vi "Export dat - I-V.vi"(8 "Error In":errorcluster, 9 "Workspace":path, 11 "IV measurement":T1={"Name"="", "Comment"="", "Time"=timestamp(0 s since 1904-01-01), "Folder"=path "", "IV properties"={"T"=0.0, "Vstart"=-0.5, "Vstop"=0.5, "Vpoints"=10.0, "Settling"=0.01, "I limit"=0.1, "Log mapping"=FALSE, "Averaging"=0.0}, "GUID"=""} {"IV properties"."Settling" min=0.0 max=65535.0}) -> (0 "Error Out":errorcluster)   [LabVIEW 2019]
doc: "Handles export of a I-V measurement to a .dat file, displays a GUI window"
uses:
  Type defs/IV measurement Type Def.ctl
  Type defs/IV properties Type Def.ctl
  <vilib>/Utility/sysdir.llb/System Directory Type.ctl
  <vilib>/Utility/file.llb/Write Delimited Spreadsheet (string).vi
  <vilib>/Utility/file.llb/Write Delimited Spreadsheet (DBL).vi
panel:
  out "String":string
  in  "Path":path caption="Export file as:"
  in  "Export":bool
  in  "Cancel":bool
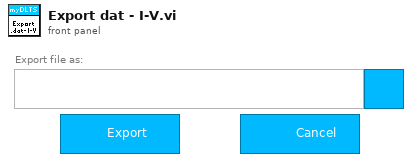
[diagram p1: front panel]
types:
  T1 = typedef "IV measurement Type Def.ctl" = cluster{"Name":string, "Comment":string, "Time":timestamp, "Folder":path, "IV properties":T2, "GUID":string}
  T2 = typedef "IV properties Type Def.ctl" = cluster{"T":dbl[unit], "Vstart":dbl[unit], "Vstop":dbl[unit], "Vpoints":dbl, "Settling":dbl[unit], "I limit":dbl[unit], "Log mapping":bool, "Averaging":dbl}
  T3 = enum32{"existing file", "new file", "new or existing file", "existing dir", "new dir", "new or existing dir", "existing file (use LLBs)", "new file (use LLBs)", "new or existing file (use LLBs)", "new or existing file or directory (use LLBs)", "existing dir (use LLBs)", "new dir (use LLBs)", "new or existing dir (use LLBs)", "existing file or dir", "new file or dir", "new or existing file or dir", "existing file or dir (use LLBs)", "new file or dir (use LLBs)"}
  T4 = typedef "System Directory Type.ctl" = i32
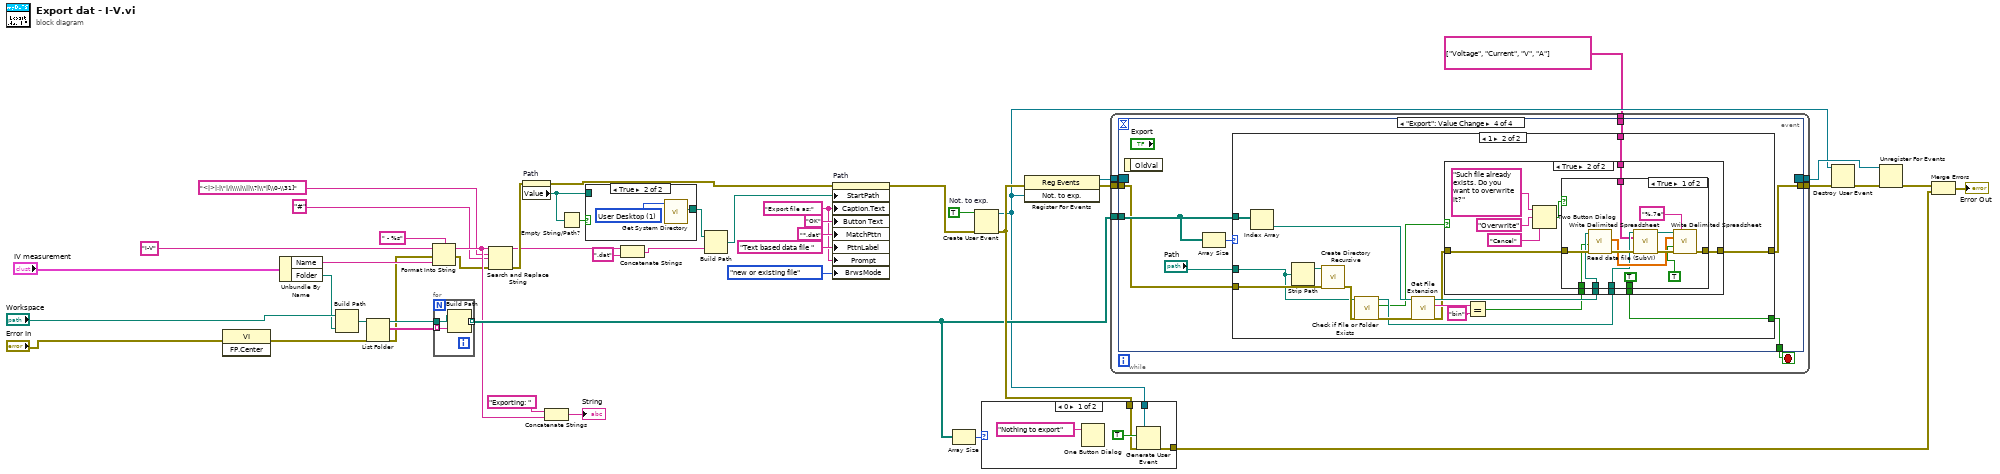
[diagram p0: block diagram]
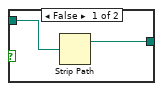
[diagram p2: hidden frame]
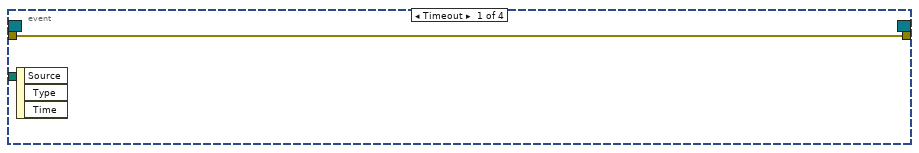
[diagram p4: hidden frame]
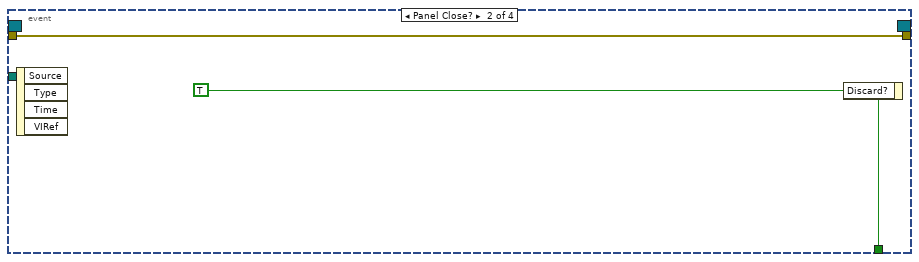
[diagram p5: hidden frame]
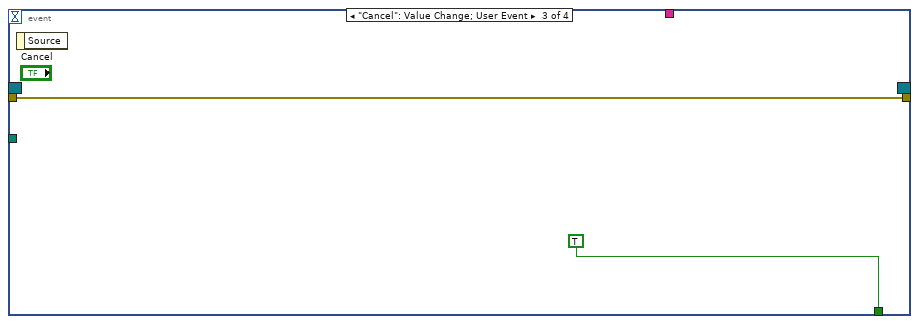
[diagram p6: hidden frame]
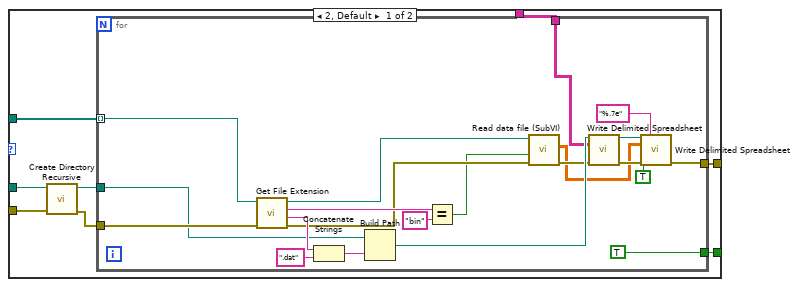
[diagram p7: hidden frame]
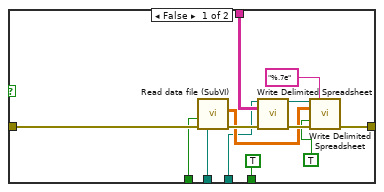
[diagram p8: hidden frame]
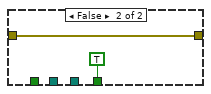
[diagram p9: hidden frame]
diagram:
  w15 = "Export file as:"
  w45 = TRUE  # Not. to exp.
  n1 = invoke class="VI" method="FP.Center"(error in="Error In") -> (error out=w3:errorcluster)  [unwired: 2 in, 2 out]
  n2 = Unbundle By Name("IV measurement") -> ("Name"=w10:string, "Folder"=w20:path)
  n3 = Build Path(base path="Workspace", name or relative path=w20) -> (appended path=w13:path)
  n4 = List Folder(path=w13, error in=w3) -> (path out=w12:path, filenames=w19:string[], error out=w5:errorcluster)  [unwired: 2 in, 1 out]
  n5 = Format Into String(format string=" - %s", initial string="I-V", error in=w5, w10) -> (resulting string=w32:string, error out=w9:errorcluster)
  n6 = for {
    tunnel: w12 -> [w50]
    tunnel: [w49] -> w40 mode=indexing
    tunnel: w19 -> [w48] mode=indexing
    n7 = Build Path(base path=w50, name or relative path=w48) -> (appended path=w49:path)
  }
  n8 = Search and Replace String(input string=w32, search string="<|>|:|\"|/|\\\\|\\||\\?|\\*|[\\0-\\31]", replace string="#" ("replace string (\"\")"), error in=w9) -> (result string=w8:string, error out=w11:errorcluster)  [unwired: 4 in, 2 out]
  n9 = property on="Path" class="Path"(error in=w11) -> (error out=w21:errorcluster, "Value"=w27:path)  [unwired: 1 in, 1 out]
  n10 = Concatenate Strings("Exporting: " ("string"), w32) -> (→"String":string)
  n11 = Empty String/Path?(string/path=w27) -> (empty?=w28:bool)
  n12 = case shown="True" w28 {
    tunnel: w27 -> [w52 _]
    tunnel: [w51 w53] -> w23
    frame False {
      n13 = Strip Path(path=w52) -> (stripped path=w51:path)  [unwired: 1 out]
    }
    frame True {
      w54 = T4 1 items=["User Home"=0, "User Desktop"=1, "User Documents"=2, "User Application Data"=3, "User Preferences"=4, "User Temporary"=5, "Public Documents"=6, "Public Application Data"=7, "Public Preferences"=8, "Public Cache"=13, "System Core Libraries"=9, "System Installed Libraries"=10, "Application Files"=11, "Boot Volume Root"=12] ("system directory type")
      n14 = call <vilib>:"Get System Directory.vi"("system directory type"=w54) -> ("system directory"=w53:path)  [unwired: 10 in]
    }
  }
  n15 = Concatenate Strings(w8, ".dat" ("string")) -> (w7:string)
  n16 = Build Path(base path=w23, name or relative path=w7) -> (appended path=w22:path)
  n17 = property on="Path" class="Path"(error in=w21, "StartPath"=w22, "Caption.Text"=w15, "Button Text"="OK", "MatchPttn"="*.dat", "PttnLabel"="Text based data file ", "Prompt"=w15, "BrwsMode"=T3."new or existing file" ("Browse Options:Selection Mode")) -> (error out=w42:errorcluster)  [unwired: 1 in, 1 out]
  n18 = Array Size(array=w40) -> (size(s)=w46:i32)
  n19 = Create User Event(user event datatype=w45, error in=w42) -> (user event=w36:refnum<user-event>, error out=w41:errorcluster)
  n20 = case shown="0" w46 {
    tunnel: w36 -> [w58 _]
    tunnel: w41 -> [w56 w60]
    tunnel: [w55 w60] -> w33
    frame 0 {
      n21 = One Button Dialog(message="Nothing to export") -> ()  [unwired: 1 in, 1 out]
      n22 = Generate User Event(user event=w58, event data cluster=TRUE ("event data"), error in=w56) -> (error out=w55:errorcluster)  [unwired: 1 in, 1 out]
    }
    frame 1, Default {
    }
  }
  n23 = register-events(error in=w41, w36) -> (reference out=w43:refnum<event-registration>, error out=w44:errorcluster)  [unwired: 1 in]
  n24 = while {
    tunnel: w44 -> [w67]
    tunnel: [w66] -> w39
    tunnel: w40 -> [w64]
    tunnel: w43 -> [w63]
    tunnel: [w62] -> w37
    tunnel: string[][] [["Voltage", "Current"], ["V", "A"]] ("2D data") -> [w61]
    stop <- w65 stop-if-true
    n25 = event shown="[3] \"Export\": Value Change" {
      selector: w63 -> [_ _ _ _]
      dyn-events: [_ _ _ _] -> w62
      timeout: _ -> [_ _ _ _]
      tunnel: w67 -> [w68 w69 w71 w76]
      tunnel: [w68 w69 w71 w75] -> w66
      tunnel: [_ w70 TRUE ("Discard?") w74] -> w65
      tunnel: w64 -> [_ _ _ w79]
      tunnel: w61 -> [_ _ _ w73]
      event Timeout {
        n26 = event-data() -> ()  [unwired: 1 in, 3 out]
      }
      event Panel Close? {
        w70 = TRUE ("Discard?")
        n27 = event-data() -> ()  [unwired: 1 in, 4 out]
        n28 = event-data("Discard?"=w70) -> ()  [unwired: 1 in, 1 out]
      }
      event "Cancel": Value Change; User Event {
        n29 = event-data() -> ()  [unwired: 1 in, 1 out]
      }
      event "Export": Value Change {
        n30 = event-data() -> ()  [unwired: 1 in, 1 out]
        n31 = Array Size(array=w79) -> (size(s)=w78:i32)
        n32 = case shown="1" w78 {
          tunnel: [w87 w115] -> w74
          tunnel: w76 -> [w84 w120]
          tunnel: w79 -> [w86 w119]
          tunnel: "Path" -> [w83 w117]
          tunnel: [w85 w116] -> w75
          tunnel: w73 -> [w80 w109]
          frame 2, Default {
            n33 = call <vilib>:"Create Directory Recursive.vi"("error in (no error)"=w84, "directory"=w83) -> ("error out"=w82:errorcluster, "directory copy"=w81:path)  [unwired: 3 in, 1 out]
            n34 = for {
              tunnel: [TRUE] -> w87
              tunnel: w86 -> [w105] mode=indexing
              tunnel: [w91] -> w85
              tunnel: w82 -> [w101]
              tunnel: w81 -> [w100]
              tunnel: w80 -> [w88]
              n35 = call <vilib>:"Get File Extension.vi"("error in (no error)"=w101, "file"=w105) -> ("error out"=w95:errorcluster, "filename without extension"=w103:string, "lowercase file extension"=w108:string, "dup file"=w96:path)  [unwired: 5 in, 1 out]
              n36 = Concatenate Strings(w103, ".dat" ("string")) -> (w104:string)
              n37 = Build Path(base path=w100, name or relative path=w104) -> (appended path=w93:path)
              n38 = Equal?(x=w108, y="bin") -> (x = y?=w94:bool)
              n39 = call "Read data file (SubVI).vi"("error in"=w95, "Binary"=w94, "file path in"=w96) -> ("error out"=w90:errorcluster, "2D data"=w89:dbl[][])  [unwired: 6 in, 1 out]
              n40 = call-poly <vilib>:"Write Delimited Spreadsheet.vi"("file path (dialog if empty)"=w93, "2D data"=w88, "error in (no error)"=w90) -> ("new file path (Not A Path if cancelled)"=w92:path, "error out"=w98:errorcluster)  [unwired: 11 in]
              n41 = call-poly <vilib>:"Write Delimited Spreadsheet.vi"("file path (dialog if empty)"=w92, "format (%.3f)"="%.7e", "2D data"=w89, "append to file? (new file:F)"=TRUE, "error in (no error)"=w98) -> ("error out"=w91:errorcluster)  [unwired: 9 in, 1 out]
            }
          }
          frame 1 {
            n42 = Index Array(array=w119) -> (element=w118:path)  [unwired: 1 in]
            n43 = Strip Path(path=w117) -> (stripped path=w122:path)  [unwired: 1 out]
            n44 = call <vilib>:"Create Directory Recursive.vi"("error in (no error)"=w120, "directory"=w122) -> ("error out"=w121:errorcluster)  [unwired: 3 in, 2 out]
            n45 = call <vilib>:"Check if File or Folder Exists.vi"("error in (no error)"=w121, "path"=w117) -> ("error out"=w123:errorcluster, "file or folder exists?"=w110:bool, "dup path"=w114:path)  [unwired: 7 in]
            n46 = call <vilib>:"Get File Extension.vi"("error in (no error)"=w123, "file"=w118) -> ("error out"=w111:errorcluster, "lowercase file extension"=w125:string, "dup file"=w113:path)  [unwired: 5 in, 2 out]
            n47 = Equal?(x=w125, y="bin") -> (x = y?=w112:bool)
            n48 = case shown="True" w110 {
              tunnel: [w131 w149] -> w116
              tunnel: [TRUE w148] -> w115
              tunnel: w111 -> [w129 w143]
              tunnel: w114 -> [w126 w142]
              tunnel: w113 -> [w127 w141]
              tunnel: w112 -> [w128 w140]
              tunnel: w109 -> [w130 w139]
              frame False {
                n49 = call "Read data file (SubVI).vi"("error in"=w129, "Binary"=w128, "file path in"=w127) -> ("error out"=w134:errorcluster, "2D data"=w133:dbl[][])  [unwired: 6 in, 1 out]
                n50 = call-poly <vilib>:"Write Delimited Spreadsheet.vi"("file path (dialog if empty)"=w126, "2D data"=w130, "error in (no error)"=w134) -> ("new file path (Not A Path if cancelled)"=w135:path, "error out"=w137:errorcluster)  [unwired: 11 in]
                n51 = call-poly <vilib>:"Write Delimited Spreadsheet.vi"("file path (dialog if empty)"=w135, "format (%.3f)"="%.7e", "2D data"=w133, "append to file? (new file:F)"=TRUE, "error in (no error)"=w137) -> ("error out"=w131:errorcluster)  [unwired: 9 in, 1 out]
              }
              frame True {
                n52 = Two Button Dialog(message="Such file already exists. Do you want to overwrite it?", 1:"Cancel" ("F button name (\"Cancel\")"), 2:"Overwrite" ("T button name (\"OK\")")) -> (T button?=w144:bool)
                n53 = case shown="True" w144 {
                  tunnel: [w155 w163] -> w149
                  tunnel: [TRUE TRUE] -> w148
                  tunnel: w143 -> [w156 w163]
                  tunnel: w142 -> [w154 _]
                  tunnel: w141 -> [w153 _]
                  tunnel: w140 -> [w152 _]
                  tunnel: w139 -> [w150 _]
                  frame True {
                    n54 = call "Read data file (SubVI).vi"("error in"=w156, "Binary"=w152, "file path in"=w153) -> ("error out"=w158:errorcluster, "2D data"=w157:dbl[][])  [unwired: 6 in, 1 out]
                    n55 = call-poly <vilib>:"Write Delimited Spreadsheet.vi"("file path (dialog if empty)"=w154, "2D data"=w150, "error in (no error)"=w158) -> ("new file path (Not A Path if cancelled)"=w159:path, "error out"=w161:errorcluster)  [unwired: 11 in]
                    n56 = call-poly <vilib>:"Write Delimited Spreadsheet.vi"("file path (dialog if empty)"=w159, "format (%.3f)"="%.7e", "2D data"=w157, "append to file? (new file:F)"=TRUE, "error in (no error)"=w161) -> ("error out"=w155:errorcluster)  [unwired: 9 in, 1 out]
                  }
                  frame False {
                  }
                }
              }
            }
          }
        }
      }
    }
  }
  n57 = Destroy User Event(user event=w36, error in=w39) -> (error out=w38:errorcluster)
  n58 = Unregister For Events(event registration refnum=w37, error in=w38) -> (error out=w35:errorcluster)
  n59 = Merge Errors(w35, w33) -> (→"Error Out":errorcluster)
